vi "SubVI 1.vi"() -> ()   [LabVIEW 2018]
panel:
  in  "Close SubVI":bool
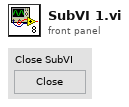
[diagram p1: front panel]
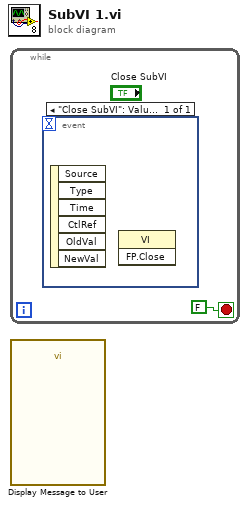
[diagram p0: block diagram]
diagram:
  n1 = while {
    stop <- FALSE stop-if-true
    n2 = event shown="[0] \"Close SubVI\": Value Change" {
      selector: _ -> [_]
      dyn-events: _ -> [_]
      timeout: _ -> [_]
      event "Close SubVI": Value Change {
        n3 = event-data() -> ()  [unwired: 1 in, 6 out]
        n4 = invoke class="VI" method="FP.Close"() -> ()  [unwired: 3 in, 3 out]
      }
    }
  }
  n5 = call "Display Message to User"() -> ()  [unwired: 10 in, 2 out]
